vi "disconnect.vi"(8 "error in (no error)":errorcluster, 11 "TCPClient in":refnum<class "TCPClient.lvclass">) -> (0 "error out":errorcluster, 3 "TCPClient out":refnum<class "TCPClient.lvclass">)   [LabVIEW 2016, in "TCPClient.lvclass"]
uses:
  TCPClient.lvclass
  C:/Users/aanania/Documents/ts_monochromator_windows/ts_labview_tcp/TCPCommunicator/TCPCommunicator.lvclass
  TCPCommunicator/TCPCommunicator.lvclass/TCPCommunicator.ctl
  TCPCommunicator/TCPCommunicator.lvclass
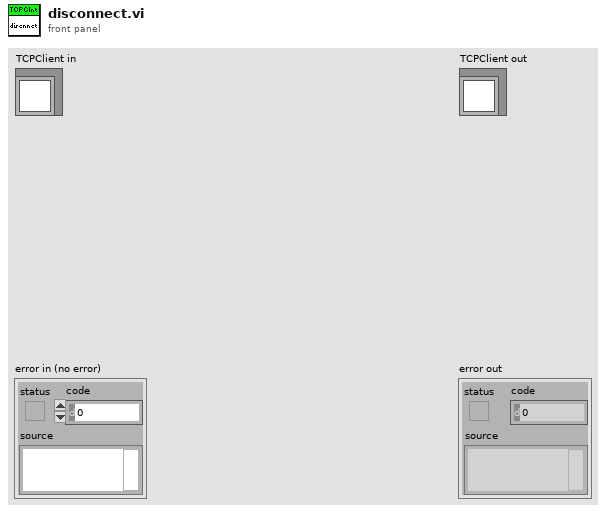
[diagram p1: front panel]
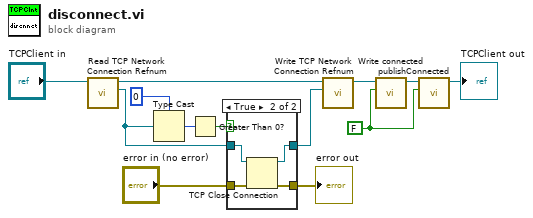
[diagram p0: block diagram]
diagram:
  w2 = FALSE ("connected")
  n1 = call-dynamic "Read TCP Network Connection Refnum.vi"("TCPCommunicator in"="TCPClient in") -> ("TCP Network Connection Refnum"=w10:refnum<k5>, "TCPCommunicator out"=w9:refnum<class "TCPClient.lvclass">)  [unwired: 8 in, 1 out]
  n2 = Type Cast(type=0, x=w10) -> (*(type *) &x=w13:i32)
  n3 = Greater Than 0?(x=w13) -> (x > 0?=w11:bool)
  n4 = case shown="True" w11 {
    tunnel: w10 -> [w14 w19]
    tunnel: "error in (no error)" -> [w15 w18]
    tunnel: [w14 w17] -> w8
    tunnel: [w15 w16] -> w4
    frame False {
    }
    frame True {
      n5 = TCP Close Connection(connection ID=w19, error in (no error)=w18) -> (connection ID out=w17:refnum<k5>, error out=w16:errorcluster)  [unwired: 1 out]
    }
  }
  "error out" <- w4
  n6 = call-dynamic "Write TCP Network Connection Refnum.vi"("TCP Network Connection Refnum"=w8, "TCPCommunicator in"=w9) -> ("TCPCommunicator out"=w7:refnum<class "TCPClient.lvclass">)  [unwired: 8 in, 1 out]
  n7 = call "Write connected.vi"("connected"=w2, "TCPCommunicator in"=w7) -> ("TCPCommunicator out"=w3:refnum<class "TCPClient.lvclass">)  [unwired: 8 in, 1 out]
  n8 = call-dynamic "publishConnected.vi"("Connected"=w2, "TCPCommunicator in"=w3) -> ("TCPCommunicator out"=→"TCPClient out":refnum<class "TCPClient.lvclass">)  [unwired: 8 in, 1 out]
